vi "thorlabs_connect.vi"(8 "error in (no error)":errorcluster, 10 "Serial":string, 11 "thorlabs_panel in":refnum<class "thorlabs_panel.lvclass">) -> (0 "error out":errorcluster, 3 "thorlabs_panel out":refnum<class "thorlabs_panel.lvclass">)   [LabVIEW 2015, in "thorlabs_panel.lvclass"]
uses:
  thorlabs_panel.lvclass
  thorlabs_class/thorlabs_kinesis.lvclass
  thorlabs_class/thorlabs_kinesis.lvclass/thorlabs_kinesis.ctl
  thorlabs_panel.lvclass/thorlabs_panel.ctl
  UI/panel_class/panel.lvclass
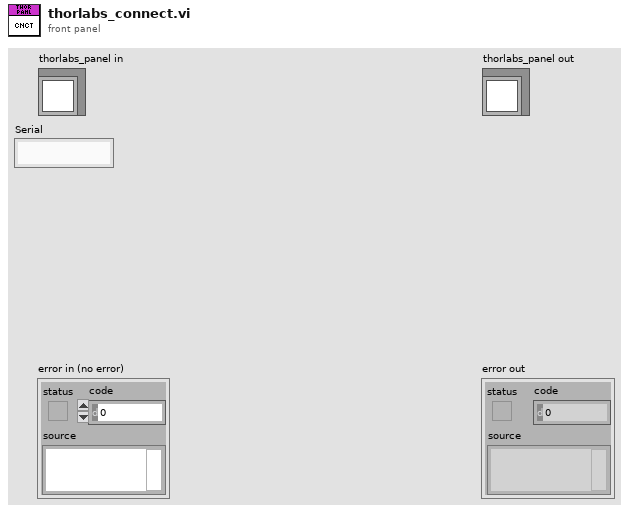
[diagram p1: front panel]
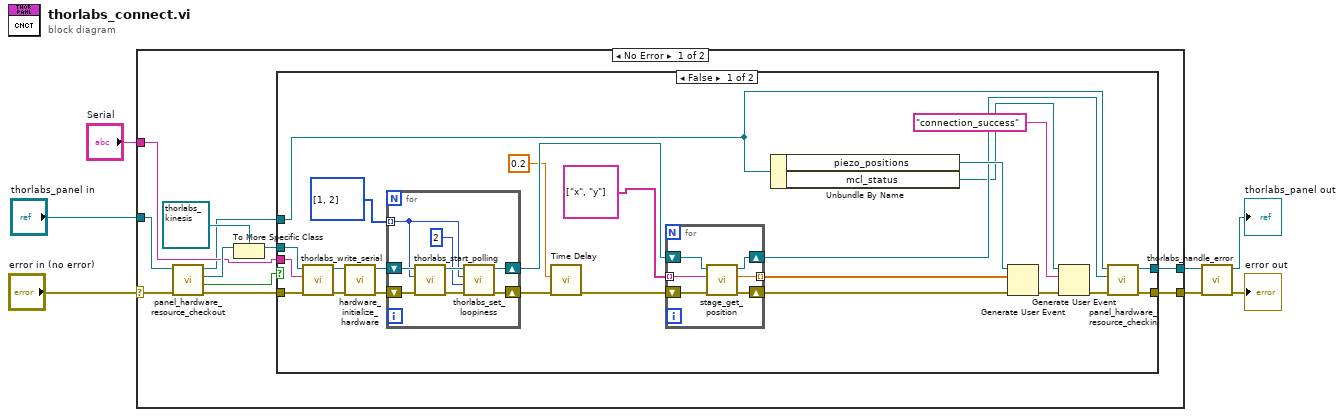
[diagram p0: block diagram]
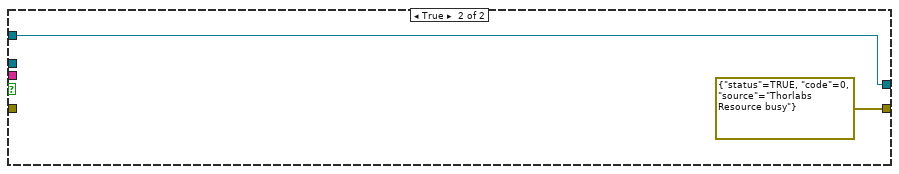
[diagram p2: hidden frame]
diagram:
  n1 = case shown="No Error" "error in (no error)" {
    selector: "error in (no error)" -> [w17 w60]
    tunnel: [w8 w60] -> w4
    tunnel: [w9 w59] -> w3
    tunnel: "thorlabs_panel in" -> [w18 w59]
    tunnel: "Serial" -> [w13 _]
    frame No Error {
      n2 = call "panel_hardware_resource_checkout.vi"("error in (no error)"=w17, "panel in"=w18) -> ("error out"=w12:errorcluster, "timed out?"=w11:bool, "hardware.lvclass"=w16:refnum<class "hardware.lvclass">, "panel out"=w10:refnum<class "thorlabs_panel.lvclass">)  [unwired: 6 in]
      n3 = To More Specific Class(target class=refnum<class "thorlabs_kinesis.lvclass"> refnum ("thorlabs_kinesis.lvclass"), reference=w16) -> (specific class reference=w14:refnum<class "thorlabs_kinesis.lvclass">)  [unwired: 1 in, 1 out]
      n4 = case shown="False" w11 {
        tunnel: w14 -> [w42 _]
        tunnel: w13 -> [w41 _]
        tunnel: w12 -> [w40 _]
        tunnel: w10 -> [w29 w57]
        tunnel: [w37 w57] -> w9
        tunnel: [w36 errorcluster {"status"=TRUE, "code"=0, "source"="Thorlabs Resource busy"} ("error out")] -> w8
        frame False {
          n5 = call "thorlabs_write_serial.vi"("error in (no error)"=w40, "serial"=w41, "thorlabs_kinesis in"=w42) -> ("error out"=w38:errorcluster, "thorlabs_kinesis out"=w39:refnum<class "thorlabs_kinesis.lvclass">)  [unwired: 7 in]
          n6 = call-dynamic "hardware_initialize_hardware.vi"("error in (no error)"=w38, "thorlabs_kinesis in"=w39) -> ("error out"=w35:errorcluster, "thorlabs_kinesis out"=w34:refnum<class "thorlabs_kinesis.lvclass">)  [unwired: 8 in]
          n7 = for {
            shift-right: [w53] -> w32
            shift-left: w35 -> [w56]
            tunnel: i32[] [1, 2] -> [w50] mode=indexing
            shift-right: [w51] -> w33
            shift-left: w34 -> [w55]
            n8 = call "thorlabs_start_polling.vi"("error in (no error)"=w56, "channel"=w50, "thorlabs_kinesis in"=w55) -> ("error out"=w54:errorcluster, "thorlabs_kinesis out"=w52:refnum<class "thorlabs_kinesis.lvclass">)  [unwired: 7 in]
            n9 = call "thorlabs_set_loopiness.vi"("error in (no error)"=w54, "PositionControlMode"=i16 2, "channel"=w50, "thorlabs_kinesis in"=w52) -> ("error out"=w53:errorcluster, "thorlabs_kinesis out"=w51:refnum<class "thorlabs_kinesis.lvclass">)  [unwired: 6 in]
          }
          n10 = call "Time Delay"("error in (no error)"=w32, "Delay Time (s)"=0.2) -> ("error out"=w30:errorcluster)  [unwired: 9 in]
          n11 = for {
            tunnel: string[] ["x", "y"] -> [w46] mode=indexing
            tunnel: [w45] -> w27 mode=indexing
            shift-right: [w44] -> w26
            shift-left: w30 -> [w47]
            shift-right: [w43] -> w25
            shift-left: w33 -> [w48]
            n12 = call-dynamic "stage_get_position.vi"("error in (no error)"=w47, "Stage Name"=w46, "Stage in"=w48) -> ("error out"=w44:errorcluster, "Position"=w45:dbl, "Stage out"=w43:refnum<class "thorlabs_kinesis.lvclass">)  [unwired: 6 in]
          }
          n13 = Unbundle By Name(w29) -> ("piezo_positions"=w28:refnum<user-event>, "mcl_status"=w23:refnum<user-event>)
          n14 = Generate User Event(user event=w28, event data cluster=w27, error in=w26) -> (error out=w24:errorcluster)  [unwired: 1 in, 1 out]
          n15 = Generate User Event(user event=w23, event data cluster="connection_success" ("event data"), error in=w24) -> (error out=w21:errorcluster)  [unwired: 1 in, 1 out]
          n16 = call "panel_hardware_resource_checkin.vi"("error in (no error)"=w21, "hardware.lvclass"=w25, "panel in"=w29) -> ("error out"=w36:errorcluster, "panel out"=w37:refnum<class "thorlabs_panel.lvclass">)  [unwired: 7 in]
        }
        frame True {
        }
      }
    }
    frame Error {
    }
  }
  n17 = call "thorlabs_handle_error.vi"("error in (no error)"=w4, "thorlabs_panel in"=w3) -> ("error out"=→"error out":errorcluster, "thorlabs_panel out"=→"thorlabs_panel out":refnum<class "thorlabs_panel.lvclass">)  [unwired: 8 in]
